vi "rethinkdb_msg_hmac.vi"(7 "blocksize (SHA256=64)":i32=64, 10 "message":string="The quick brown fox jumps over the lazy dog", 11 "key":string="key") -> (3 "sha-256 hash":u32[](array[numeric]) format="%08x")   [LabVIEW 2017]
panel:
  # "f7bc83f4 30538424 b13298e6 aa6fb143 ef4d59a1 49461759 97479dbc 2d1a3cd8"
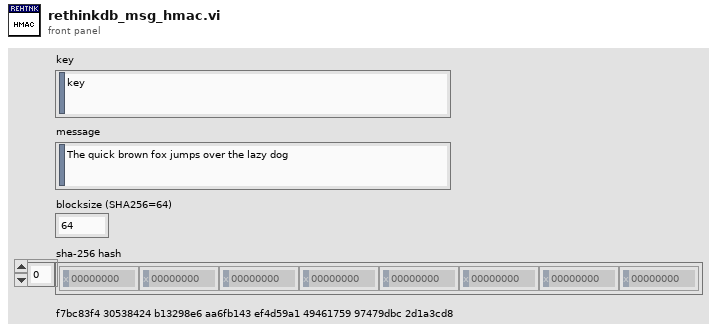
[diagram p1: front panel]
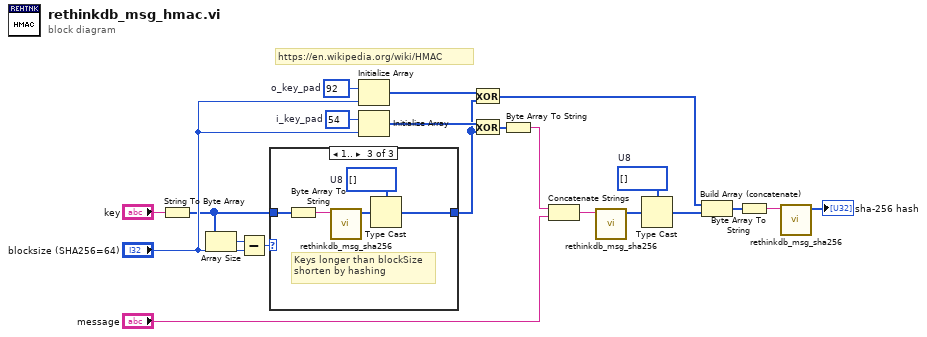
[diagram p0: block diagram]
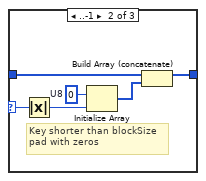
[diagram p3: hidden frame]
diagram:
  w8 = u8[] []  # U8
  w18 = u8 92  # o_key_pad
  w19 = u8 54  # i_key_pad
  # "https://en.wikipedia.org/wiki/HMAC"
  n1 = String To Byte Array(string="key") -> (unsigned byte array=w2:u8[])
  n2 = Array Size(array=w2) -> (size(s)=w1:i32)
  n3 = Subtract(x=w1, y="blocksize (SHA256=64)") -> (x-y=w20:i32)
  n4 = case shown="1.." w20 {
    selector: w20 -> [_ w28 _]
    tunnel: w2 -> [w22 w23 w33]
    tunnel: [w22 w25 w31] -> w14
    frame 0 {
      # "Same size"
    }
    frame ..-1 {
      w26 = u8 0  # U8
      # "Key shorter than blockSize\npad with zeros"
      n5 = Absolute Value(x=w28) -> (abs(x)=w27:i32)
      n6 = Initialize Array(w26, w27) -> (w24:u8[])
      n7 = Build Array (concatenate)(w23, w24) -> (w25:u8[])
    }
    frame 1.. {
      w30 = u8[] []  # U8
      # "Keys longer than blockSize\nshorten by hashing"
      n8 = Byte Array To String(unsigned byte array=w33) -> (string=w29:string)
      n9 = call "rethinkdb_msg_sha256.vi"("string"=w29) -> ("sha-256 hash"=w32:u32[])  [unwired: 10 in]
      n10 = Type Cast(type=w30, x=w32) -> (*(type *) &x=w31:u8[])
    }
  }
  n11 = Initialize Array(w18, "blocksize (SHA256=64)") -> (w15:u8[])
  n12 = Initialize Array(w19, "blocksize (SHA256=64)") -> (w16:u8[])
  n13 = Exclusive Or(1:w14, 2:w15) -> (0:w9:u8[])
  n14 = Exclusive Or(1:w14, 2:w16) -> (0:w13:u8[])
  n15 = Byte Array To String(unsigned byte array=w13) -> (string=w12:string)
  n16 = Concatenate Strings(w12, "message") -> (w10:string)
  n17 = call "rethinkdb_msg_sha256.vi"("string"=w10) -> ("sha-256 hash"=w7:u32[])  [unwired: 10 in]
  n18 = Type Cast(type=w8, x=w7) -> (*(type *) &x=w6:u8[])
  n19 = Build Array (concatenate)(w9, w6) -> (w5:u8[])
  n20 = Byte Array To String(unsigned byte array=w5) -> (string=w4:string)
  n21 = call "rethinkdb_msg_sha256.vi"("string"=w4) -> ("sha-256 hash"=→"sha-256 hash":u32[])  [unwired: 10 in]
